vi "pulsteller.vi"() -> ()   [LabVIEW 2019]
uses:
  <vilib>/myRIO/Common/Instrument Driver Framework/myRIO v1.0/Encoder/typedefs/Encoder Signal Mode.ctl
  <vilib>/myRIO/Instrument Drivers/Onboard IO/Encoder/typedefs/Encoder Reference.ctl
  <vilib>/myRIO/Common/Instrument Driver Framework/Utilities/typedefs/myRIO Generic Hardware Reference.ctl
  <vilib>/myRIO/Common/Instrument Driver Framework/Utilities/typedefs/Hardware Version Enum.ctl
  <vilib>/myRIO/Common/Instrument Driver Framework/Utilities/typedefs/myRIO v1.0 Reference.ctl
  <vilib>/myRIO/Common/Instrument Driver Framework/Utilities/typedefs/Generic FPGA Reference.ctl
  <vilib>/myRIO/Common/Instrument Driver Framework/myRIO v1.0/Encoder/typedefs/Encoder Channels Enum.ctl
  <vilib>/myRIO/Common/Instrument Driver Framework/myRIO v1.0/Encoder/typedefs/Encoder Configuration v1.0.ctl
  <vilib>/userDefined/High Color/nirio_resource_hc.ctl
  <vilib>/myRIO/Common/Instrument Driver Framework/Utilities/vis/Is FPGA Ref Available.vi
  <vilib>/myRIO/Common/Instrument Driver Framework/myRIO v1.0/Encoder/vis/myRIO v1.1 Open Encoder.vi
  <vilib>/myRIO/Instrument Drivers/Onboard IO/Encoder/vis/Read.vi
  <vilib>/myRIO/Common/Instrument Driver Framework/Utilities/vis/Validate Channels.vi
  <vilib>/myRIO/Common/Instrument Driver Framework/myRIO v1.0/Encoder/vis/myRIO v1.0 Reserve Encoder.vi
  <vilib>/myRIO/Common/Instrument Driver Framework/myRIO v1.0/Encoder/vis/myRIO v1.0 Build MUX Configuration Encoder.vi
  <vilib>/myRIO/Common/Instrument Driver Framework/myRIO v1.0/Resource Manager/vis/myRIO v1.0 Reserve Channel List.vi
  <vilib>/myRIO/Common/Instrument Driver Framework/myRIO v1.0/Resource Manager/vis/myRIO v1.0 Create Configuration List.vi
  <vilib>/myRIO/Common/Instrument Driver Framework/myRIO v1.0/Resource Manager/vis/myRIO v1.0 Reserve Channel.vi
  <vilib>/myRIO/Common/Instrument Driver Framework/myRIO v1.0/Resource Manager/vis/myRIO v1.0 Unreserve Channel.vi
  <vilib>/myRIO/Common/Instrument Driver Framework/myRIO v1.0/Resource Manager/vis/myRIO v1.0 Build Mutex Name.vi
  <vilib>/Utility/VariantDataType/GetNumericInfo.vi
  <vilib>/Utility/error.llb/Error Cluster From Error Code.vi
  <vilib>/myRIO/Common/Instrument Driver Framework/myRIO v1.0/myRIO v1.1 Open.vi
  <vilib>/myRIO/Common/Instrument Driver Framework/Utilities/vis/IO Manager.vi
  <vilib>/myRIO/Common/Instrument Driver Framework/Utilities/vis/Configuration Manager.vi
  <vilib>/myRIO/Common/Instrument Driver Framework/myRIO v1.0/Resource Manager/vis/myRIO v1.0 Configure IO.vi
  <vilib>/myRIO/Common/Instrument Driver Framework/myRIO v1.0/myRIO v1.0 Close.vi
  <vilib>/myRIO/Common/Instrument Driver Framework/myRIO v1.0/Encoder/vis/myRIO v1.0 Configure Encoder.vi
  <vilib>/myRIO/Common/Instrument Driver Framework/myRIO v1.0/Encoder/vis/myRIO v1.0 Read Encoder.vi
  <vilib>/myRIO/Express VI/Onboard IO/Encoder/Encoder Express VI.xnode
  <vilib>/myRIO/Instrument Drivers/Onboard IO/Encoder/vis/myRIO Encoder Open.xnode
  <vilib>/myRIO/Common/Instrument Driver Framework/myRIO v1.0/Encoder/typedefs/Encoder Count Direction Enum.ctl
  <vilib>/myRIO/Instrument Drivers/Onboard IO/Encoder/Encoder.lvlib
  <vilib>/ptbypt/NI_PtbyPt.lvlib
panel:
  out "km/h":dbl format="%#_2g"
  out "km/h left belt":dbl(knob) scale=0.0..15.0
  out "Pulstime left":u32
  out "Counter Value left":i32
  out "km/h":dbl format="%#_2g"
  out "km/h Right belt":dbl(knob) scale=0.0..15.0
  out "Pulstime Right":u32
  in  "Reset Counter":bool
  out "Counter Value Right":i32
  in  "Stop":bool
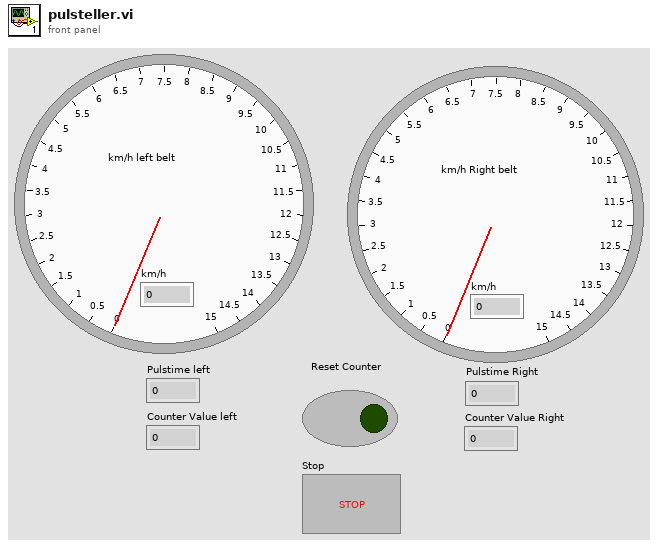
[diagram p1: front panel]
types:
  T1 = typedef "Encoder.lvlib/Encoder Reference.ctl" = cluster{"myRIO Reference":T2, "Encoder Channels Enum":T6}
  T2 = typedef "myRIO Generic Hardware Reference.ctl" = cluster{"myRIO Model":T3, "myRIO Hardware Reference":T4}
  T3 = typedef "Hardware Version Enum.ctl" = enum16{"Unknown", "myRIO-1900", "myRIO-1950", "roboRIO", "NI ELVIS RIO CM", "ELVIS III"}
  T4 = typedef "myRIO v1.0 Reference.ctl" = cluster{"Generic FPGA Reference":T5, "Allow multiple opens":bool}
  T5 = typedef "Generic FPGA Reference.ctl" = refnum<k20>
  T6 = typedef "Encoder Channels Enum.ctl" = enum16{"Not Connected", "C/ENC0", "C/ENC1", "A/ENC", "A/ENC0", "A/ENC1", "A/ENC2", "A/ENC3", "A/ENC4", "A/ENC5", "A/ENC6", "A/ENC7", "A/ENC8", "A/ENC9", "B/ENC", "B/ENC0", "B/ENC1", "B/ENC2", "B/ENC3", "B/ENC4", "B/ENC5", "B/ENC6", "B/ENC7", "B/ENC8", "B/ENC9", "DIO/ENC0", "DIO/ENC1", "DIO/ENC2", "DIO/ENC3", "DIO/ENC4"}
  T7 = typedef "Encoder Signal Mode.ctl" = enum16{"Quadrature phase signal", "Step and direction signal"}
  T8 = typedef "nirio_resource_hc.ctl" = tag
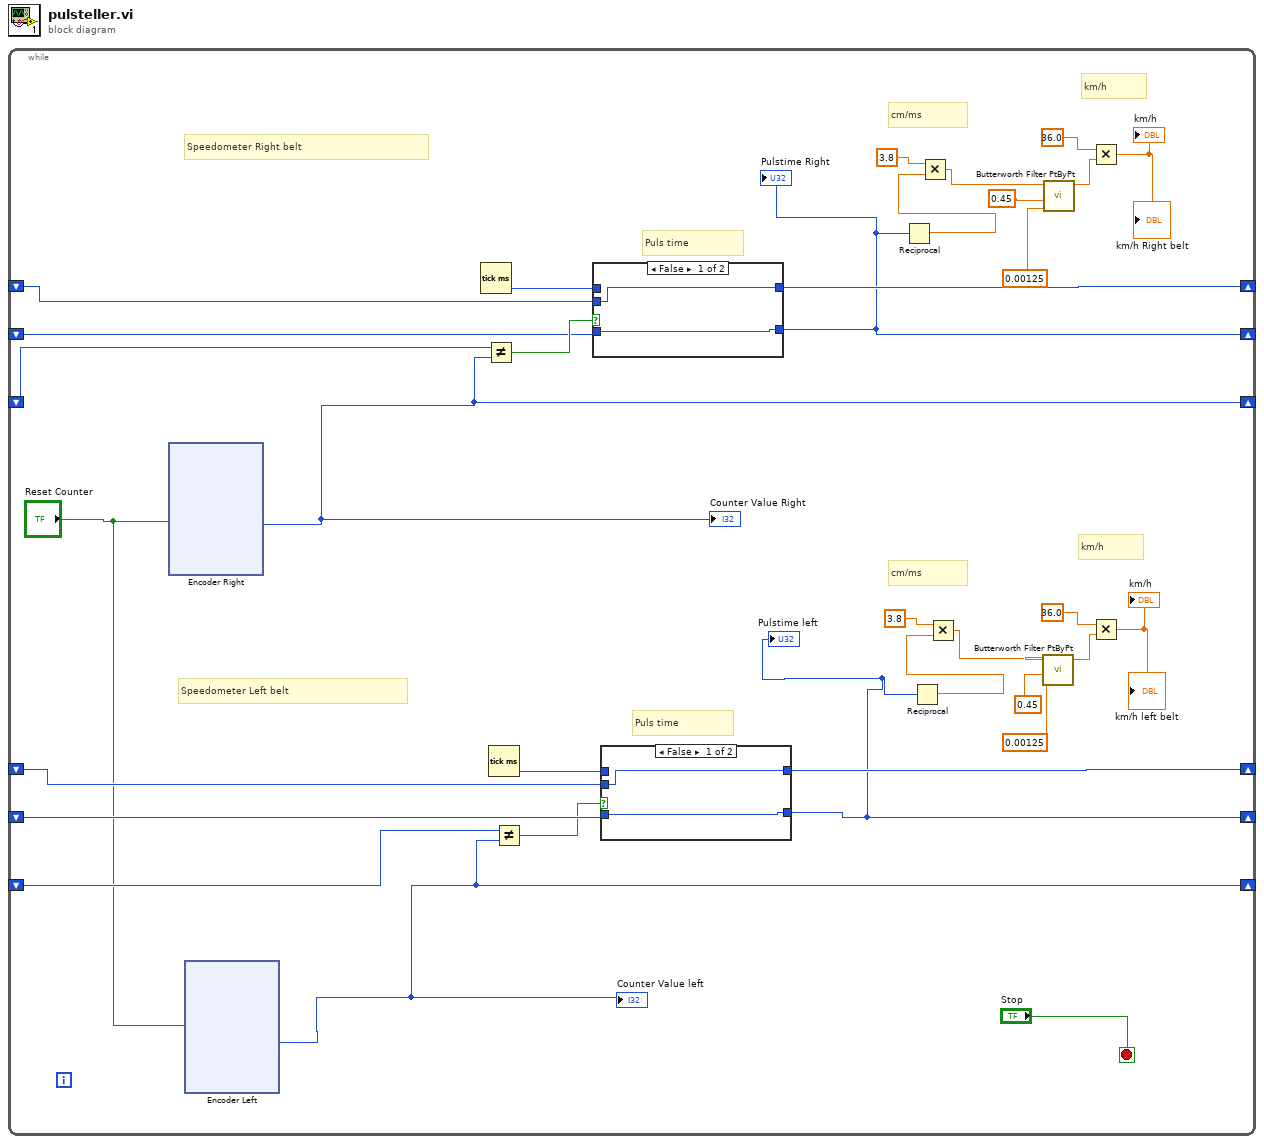
[diagram p0: block diagram]
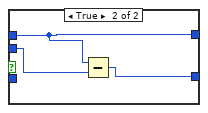
[diagram p2: hidden frame]
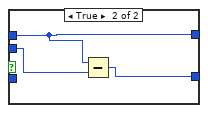
[diagram p3: hidden frame]
diagram:
  n1 = while {
    shift-right: [w2] -> _
    shift-left: _ -> [w33]
    shift-right: [w31] -> _
    shift-left: _ -> [w29]
    shift-right: [w4] -> _
    shift-left: _ -> [w28]
    shift-right: [w3] -> _
    shift-left: _ -> [w15]
    shift-right: [w7] -> _
    shift-left: _ -> [w18]
    shift-right: [w6] -> _
    shift-left: _ -> [w19]
    stop <- "Stop" stop-if-true
    # "Puls time"
    # "Puls time"
    # "km/h"
    # "cm/ms"
    # "km/h"
    # "cm/ms"
    # "Speedometer Left belt"
    # "Speedometer Right belt"
    n2 = xnode "Encoder Right"("Reset Counter"="Reset Counter") -> ("Counter Value"=w2:i32)  [unwired: 1 in, 3 out]
    "Counter Value Right" <- w2
    n3 = xnode "Encoder Left"("Reset Counter"="Reset Counter") -> ("Counter Value"=w3:i32)  [unwired: 1 in, 3 out]
    "Counter Value left" <- w3
    n4 = Tick Count (ms)() -> (millisecond timer value=w30:u32)
    n5 = Not Equal?(x=w33, y=w2) -> (x != y?=w32:bool)
    n6 = Tick Count (ms)() -> (millisecond timer value=w17:u32)
    n7 = Not Equal?(x=w15, y=w3) -> (x != y?=w16:bool)
    n8 = case shown="False" w32 {
      tunnel: [w87 w90] -> w31
      tunnel: w30 -> [_ w90]
      tunnel: w29 -> [w87 w89]
      tunnel: [w86 w88] -> w4
      tunnel: w28 -> [w86 _]
      frame False {
      }
      frame True {
        n9 = Subtract(x=w90, y=w89) -> (x-y=w88:u32)
      }
    }
    "Pulstime Right" <- w4
    n10 = case shown="False" w16 {
      tunnel: [w36 w39] -> w7
      tunnel: w17 -> [_ w39]
      tunnel: w18 -> [w36 w38]
      tunnel: [w35 w37] -> w6
      tunnel: w19 -> [w35 _]
      frame False {
      }
      frame True {
        n11 = Subtract(x=w39, y=w38) -> (x-y=w37:u32)
      }
    }
    "Pulstime left" <- w6
    n12 = Reciprocal(x=w4) -> (1/x=w27:dbl)
    n13 = Reciprocal(x=w6) -> (1/x=w8:dbl)
    n14 = Multiply(x=3.8, y=w27) -> (x*y=w26:dbl)
    n15 = Multiply(x=3.8, y=w8) -> (x*y=w1:dbl)
    n16 = call <vilib>:"Butterworth Filter PtByPt.vi"("low cutoff freq: fl"=0.00125, "high cutoff freq: fh"=0.45, "x"=w1) -> ("Filtered x"=w12:dbl)  [unwired: 6 in, 1 out]
    n17 = call <vilib>:"Butterworth Filter PtByPt.vi"("low cutoff freq: fl"=0.00125, "high cutoff freq: fh"=0.45, "x"=w26) -> ("Filtered x"=w22:dbl)  [unwired: 6 in, 1 out]
    n18 = Multiply(x=36.0, y=w22) -> (x*y=→"km/h Right belt" →"km/h":dbl)
    n19 = Multiply(x=36.0, y=w12) -> (x*y=→"km/h left belt" →"km/h":dbl)
  }
